vi "Using Temperature.vi"() -> ()   [LabVIEW 2015]
panel:
  in  "Stop Button":bool
  out "Temperature Chart":dbl(graph)
  in  "Delay Multiplier":dbl(knob) min=0.0 max=2.0 step=0.1 scale=0.0..2.0
  in  "Number of Measurements":i32
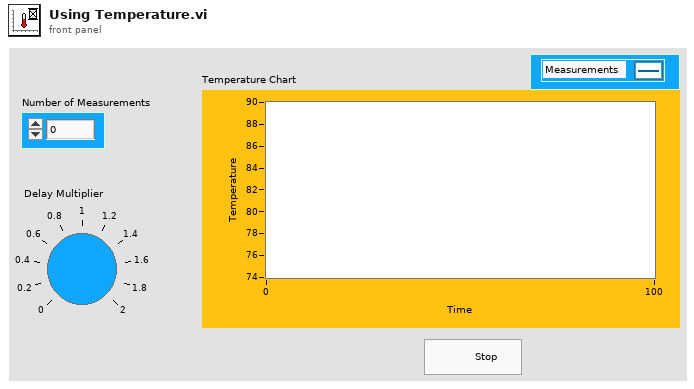
[diagram p1: front panel]
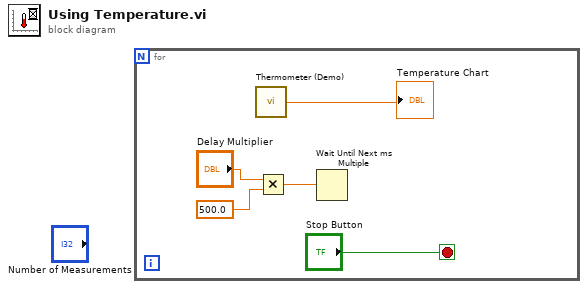
[diagram p0: block diagram]
diagram:
  n1 = for {
    stop <- "Stop Button" stop-if-true
    n2 = call "Thermometer (Demo).vi"() -> ("Temperature Value"=→"Temperature Chart":dbl)  [unwired: 1 in]
    n3 = Multiply(x="Delay Multiplier", y=500.0) -> (x*y=w3:dbl)
    n4 = Wait Until Next ms Multiple(millisecond multiple=w3) -> ()  [unwired: 1 out]
  }
